vi "Object Filter (SubVI).vi"(0 "Particle Report":T1, 1 "Box Side":cluster{"Low":u32, "High":u32}={"Low"=15, "High"=255}, 2 "Box W + L":cluster{"Low":u32, "High":u32}={"Low"=15, "High"=255}, 3 "Area":cluster{"Low":u32, "High":u32}={"Low"=15, "High"=255}) -> (4 "Bounding Box":u64, 6 "Data Valid":bool)   [LabVIEW 2020]
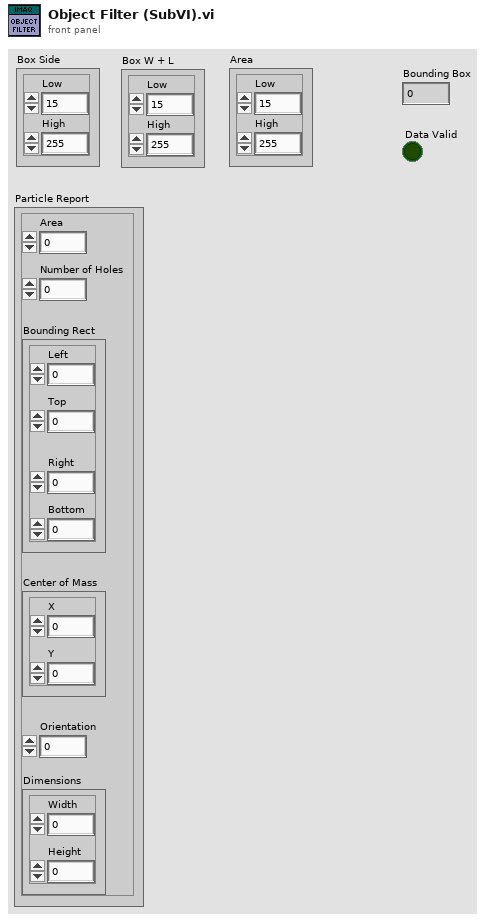
[diagram p1: front panel]
types:
  T1 = cluster{"Area":dbl, "Number of Holes":dbl, "Bounding Rect":cluster{"Left":dbl, "Top":dbl, "Right":dbl, "Bottom":dbl}, "Center of Mass":cluster{"X":dbl, "Y":dbl}, "Orientation":dbl, "Dimensions":cluster{"Width":dbl, "Height":dbl}}
  T2 = cluster{"Left":dbl, "Top":dbl, "Right":dbl, "Bottom":dbl}
  T3 = cluster{"Left":u16, "Top":u16, "Right":u16, "Bottom":u16}
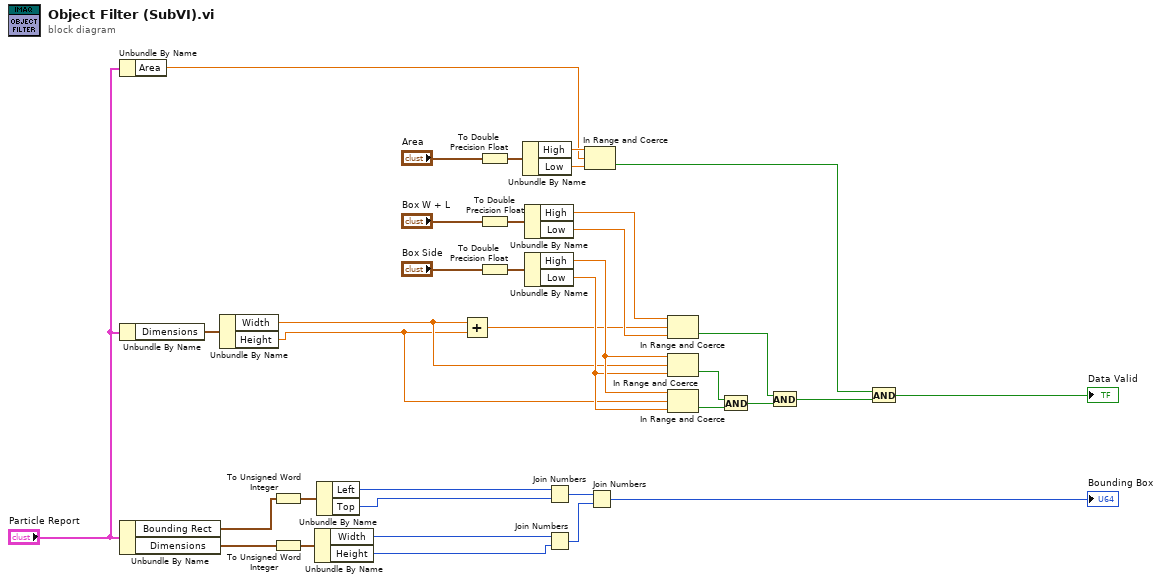
[diagram p0: block diagram]
diagram:
  n1 = Unbundle By Name("Particle Report") -> ("Area"=w13:dbl)
  n2 = Unbundle By Name("Particle Report") -> ("Dimensions"=w5:cluster{"Width":dbl, "Height":dbl})
  n3 = Unbundle By Name("Particle Report") -> ("Bounding Rect"=w31:T2, "Dimensions"=w3:cluster{"Width":dbl, "Height":dbl})
  n4 = Unbundle By Name(w5) -> ("Width"=w7:dbl, "Height"=w6:dbl)
  n5 = To Unsigned Word Integer(number=w31) -> (unsigned 16bit integer=w11:T3)
  n6 = To Unsigned Word Integer(number=w3) -> (unsigned 16bit integer=w4:cluster{"Width":u16, "Height":u16})
  n7 = Unbundle By Name(w4) -> ("Width"=w2:u16, "Height"=w1:u16)
  n8 = Unbundle By Name(w11) -> ("Left"=w30:u16, "Top"=w29:u16)
  n9 = Add(x=w7, y=w6) -> (x+y=w9:dbl)
  n10 = To Double Precision Float(number="Area") -> (double precision float=w8:cluster{"Low":dbl, "High":dbl})
  n11 = To Double Precision Float(number="Box W + L") -> (double precision float=w21:cluster{"Low":dbl, "High":dbl})
  n12 = To Double Precision Float(number="Box Side") -> (double precision float=w28:cluster{"Low":dbl, "High":dbl})
  n13 = Unbundle By Name(w8) -> ("High"=w15:dbl, "Low"=w14:dbl)
  n14 = Unbundle By Name(w21) -> ("High"=w19:dbl, "Low"=w18:dbl)
  n15 = Unbundle By Name(w28) -> ("High"=w27:dbl, "Low"=w26:dbl)
  n16 = Join Numbers(hi=w30, lo=w29) -> ((hi.lo)=w32:u32)
  n17 = Join Numbers(hi=w2, lo=w1) -> ((hi.lo)=w33:u32)
  n18 = In Range and Coerce(upper limit=w15, x=w13, lower limit=w14) -> (In Range?=w12:bool)  [unwired: 1 out]
  n19 = Join Numbers(hi=w32, lo=w33) -> ((hi.lo)=→"Bounding Box":u64)
  n20 = In Range and Coerce(upper limit=w19, x=w9, lower limit=w18) -> (In Range?=w22:bool)  [unwired: 1 out]
  n21 = In Range and Coerce(upper limit=w27, x=w7, lower limit=w26) -> (In Range?=w24:bool)  [unwired: 1 out]
  n22 = In Range and Coerce(upper limit=w27, x=w6, lower limit=w26) -> (In Range?=w23:bool)  [unwired: 1 out]
  n23 = And(x=w24, y=w23) -> (x .and. y?=w25:bool)
  n24 = And(x=w22, y=w25) -> (x .and. y?=w36:bool)
  n25 = And(x=w12, y=w36) -> (x .and. y?=→"Data Valid":bool)
